vi "test_SomeReservedSessionsRegistered_CallCloseSessions_CloseCalledForSessionsWithProperBehavior.vi"(8 "error in":errorcluster) -> (0 "error out":errorcluster, 2 "result":string, 3 "pass":bool)   [LabVIEW 2020, in "MeasurementServerTests.lvlib"]
uses:
  MeasurementServerTests.lvlib
  da6ffb6f-c1c9-4957-84dd-e9228483c454.vi
  Helpers/Fake Instrument/Fake Instrument.lvclass
  \\tsclient\C/dev/measurementlink-labview/Source/Runtime/MeasurementLink Instrument/IInstrument/IInstrument.lvclass
  Runtime/MeasurementLink Session Management/Session Reservation/Create Sessions Dispatcher.vi
  Runtime/MeasurementLink Session Management/Session Reservation/Session Reservation.lvclass
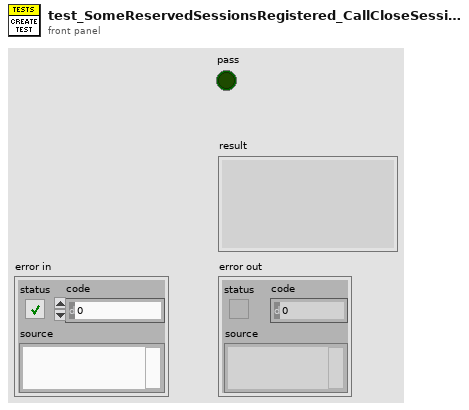
[diagram p1: front panel]
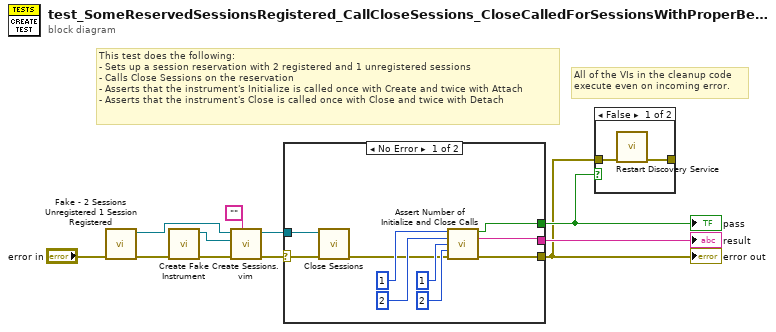
[diagram p0: block diagram]
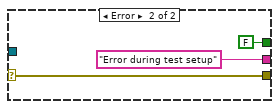
[diagram p2: hidden frame]
diagram:
  # "All of the VIs in the cleanup code\nexecute even on incoming error."
  # "This test does the following:\n- Sets up a session reservation with 2 registered and 1 unregistered sessions\n- Calls Close Sessions on the reservation\n- Asserts that the instrument's Initialize is called once with Create and twice with Attach\n- Asserts that the instrument's Close is called once with Close and twice with Detach"
  n1 = call "Fake - 2 Sessions Unregistered 1 Session Registered.vi"("error in"="error in") -> ("error out"=w7:errorcluster, "session reservation out"=w4:refnum<class "Session Reservation.lvclass">)  [unwired: 9 in]
  n2 = call "Create Fake Instrument.vi"("error in"=w7) -> ("error out"=w3:errorcluster, "fake instrument out"=w5:refnum<class "Fake Instrument.lvclass">)  [unwired: 9 in]
  n3 = call "Create Sessions.vim"("session type"="", "error in"=w3, "instrument"=w5, "session reservation in"=w4) -> ("error out"=w2:errorcluster, "session reservation out"=w1:refnum<class "Session Reservation.lvclass">)  [unwired: 4 in, 2 out]
  n4 = case shown="No Error" w2 {
    selector: w2 -> [w14 w22]
    tunnel: [w19 w22] -> w9
    tunnel: [w16 FALSE] -> w10
    tunnel: [w15 "Error during test setup" ("f")] -> w11
    tunnel: w1 -> [w12 _]
    frame No Error {
      n5 = call "Close Sessions.vi"("error in"=w14, "session reservation in"=w12) -> ("error out"=w13:errorcluster)  [unwired: 8 in, 1 out]
      n6 = call "Assert Number of Initialize and Close Calls.vi"("expected initialize-create calls"=u32 1, "expected initialize-attach calls"=u32 2, "expected close-close calls"=u32 1, "expected close-detach calls"=u32 2, "error in"=w13) -> ("pass"=w16:bool, "result"=w15:string, "error out"=w19:errorcluster)  [unwired: 8 in]
    }
    frame Error {
    }
  }
  "error out" <- w9
  "pass" <- w10
  "result" <- w11
  n7 = case shown="False" w10 {
    tunnel: w9 -> [w26 _]
    tunnel: [w25 _] -> _
    frame False {
      n8 = call "Restart Discovery Service.vi"("error in"=w26) -> ("error out"=w25:errorcluster)  [unwired: 10 in]
    }
    frame True {
    }
  }
